vi "Delete First Element.vi"(0 "Variant (Cluster) in":variant, 11 "error in (no error)":errorcluster) -> (4 "Variant (Cluster) out":variant, 6 "Name":string, 8 "element":variant, 15 "error out":errorcluster)   [LabVIEW 2017, in "Advanced Variant Tools.lvlib"]
uses:
  Advanced Variant Tools.lvlib
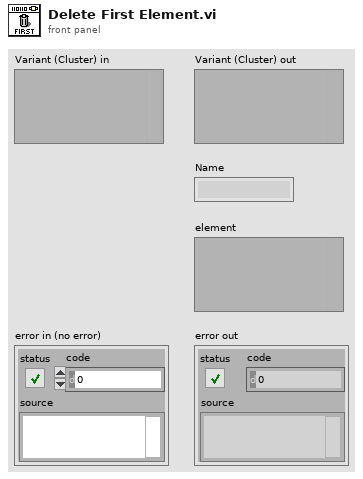
[diagram p1: front panel]
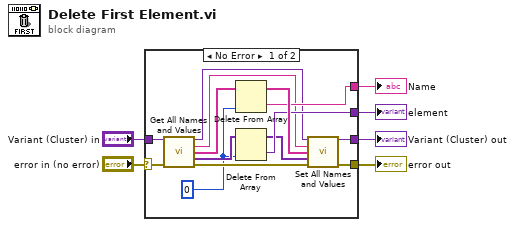
[diagram p0: block diagram]
diagram:
  n1 = case shown="No Error" "error in (no error)" {
    selector: "error in (no error)" -> [w20 w21]
    tunnel: [w18 w21] -> w5
    tunnel: [w17 w22] -> w4
    tunnel: "Variant (Cluster) in" -> [w16 w22]
    tunnel: [w13 _] -> w2
    tunnel: [w12 _] -> w1
    frame No Error {
      w9 = 0 ("index")
      n2 = call "Get All Names and Values.vi"("Variant (Cluster) In"=w16, "error in"=w20) -> ("Variant (Cluster) Out"=w7:variant, "Name"=w8:string, "Element Names"=w15:string[], "Values"=w11:variant[], "error out"=w19:errorcluster)  [unwired: 9 in]
      n3 = Delete From Array(array=w15, index=w9) -> (deleted portion=w13:string, array with subset deleted=w14:string[])  [unwired: 1 in]
      n4 = Delete From Array(array=w11, index=w9) -> (deleted portion=w12:variant, array with subset deleted=w10:variant[])  [unwired: 1 in]
      n5 = call "Set All Names and Values.vi"("Variant (Cluster) In"=w7, "Name"=w8, "Element Names"=w14, "values"=w10, "error in"=w19) -> ("Variant (Cluster) Out"=w17:variant, "error out"=w18:errorcluster)  [unwired: 9 in]
    }
    frame Error {
    }
  }
  "Variant (Cluster) out" <- w4
  "error out" <- w5
  "element" <- w1
  "Name" <- w2
